vi "NIDCPower_channel_ganging - confgure triggers waveform mode.vi"(8 "error in (no error)":errorcluster, 11 "Ganged Session in":T1) -> (0 "error out":errorcluster, 3 "Ganged Session out":T1)   [LabVIEW 2021]
uses:
  ctl/NIDCPower_channel_ganging - ctl - channel mode.ctl
  <instrlib>/niDCPower/nidcpower.llb/niDCPower Configure Digital Edge Measure Trigger With Channels.vi
  <instrlib>/niDCPower/nidcpower.llb/niDCPower Configure Digital Edge Start Trigger With Channels.vi
  ctl/NIDCPower_channel_ganging - ctl - ganged config.ctl
  ctl/NIDCPower_channel_ganging - ctl - ganged session.ctl
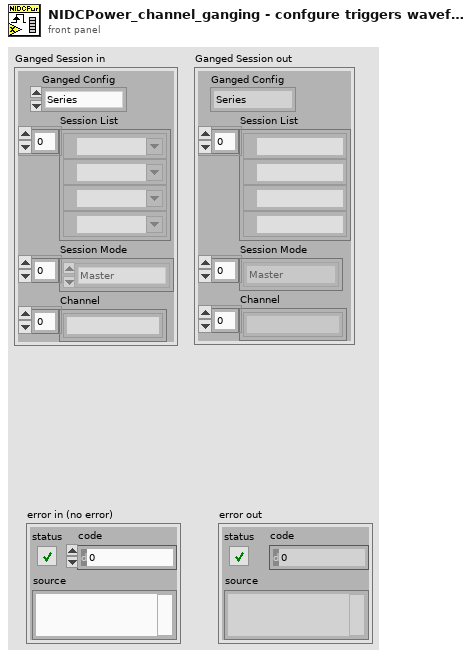
[diagram p1: front panel]
types:
  T1 = typedef "NIDCPower_channel_ganging - ctl - ganged session.ctl" = cluster{"Ganged Config":T2, "Session List":refnum<k15>[], "Session Mode":T3[], "Channel":string[]}
  T2 = typedef "NIDCPower_channel_ganging - ctl - ganged config.ctl" = enum16{"Series", "Parallel", "Manual"}
  T3 = typedef "NIDCPower_channel_ganging - ctl - channel mode.ctl" = enum16{"Master", "Slave", "Slave - Inverted"}
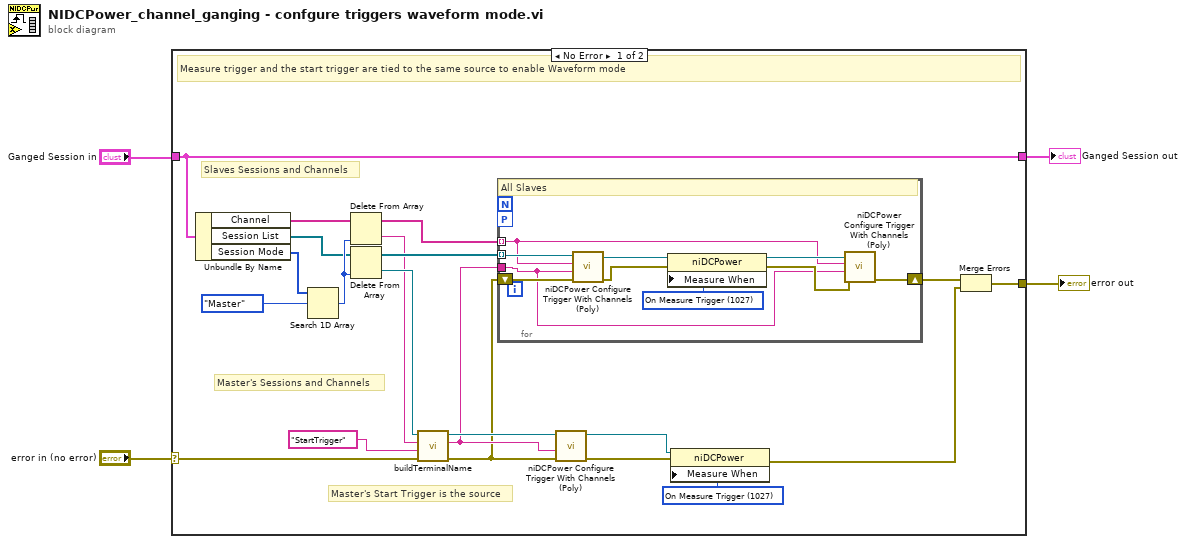
[diagram p0: block diagram]
diagram:
  n1 = case shown="No Error" "error in (no error)" {
    selector: "error in (no error)" -> [w23 w37]
    tunnel: [w9 w37] -> w4
    tunnel: "Ganged Session in" -> [w18 w36]
    tunnel: [w18 w36] -> w2
    frame No Error {
      w20 = 1027 items=["Automatically after Source Complete"=1025, "On Demand"=1026, "On Measure Trigger"=1027] ("Measurement:Advanced:Measure When")
      # "Master's Sessions and Channels"
      # "Slaves Sessions and Channels"
      # "Master's Start Trigger is the source"
      # "Measure trigger and the start trigger are tied to the same source to enable Waveform mode"
      n2 = Unbundle By Name(w18) -> ("Channel"=w14:string[], "Session List"=w13:refnum<k15>[], "Session Mode"=w6:T3[])
      n3 = Search 1D Array(1D array=w6, element=NIDCPower_channel_ganging_-_ctl_-_channel_mode."Master" ("Channel Mode")) -> (index of element=w16:i32)  [unwired: 1 in]
      n4 = Delete From Array(array=w14, index=w16) -> (deleted portion=w5:string, array with subset deleted=w15:string[])  [unwired: 1 in]
      n5 = Delete From Array(array=w13, index=w16) -> (deleted portion=w8:refnum<k15>, array with subset deleted=w17:refnum<k15>[])  [unwired: 1 in]
      n6 = call "buildTerminalName.vi"("error in (no error)"=w23, "Local Terminal Name"="StartTrigger" ("Trigger Type"), "Channel Name"=w5, "session handle"=w8) -> ("error out"=w7:errorcluster, "Fully Qualified Terminal Name"=w12:string, "session handle out"=w25:refnum<k15>)  [unwired: 5 in]
      n7 = for {
        tunnel: w15 -> [w27] mode=indexing
        tunnel: w17 -> [w28] mode=indexing
        shift-right: [w31] -> w11
        shift-left: w7 -> [w35]
        workers-P: _ -> [_]
        tunnel: w12 -> [w26]
        w32 = 1027 items=["Automatically after Source Complete"=1025, "On Demand"=1026, "On Measure Trigger"=1027] ("Measurement:Advanced:Measure When")
        # "All Slaves"
        n8 = call-poly <instrlib>:"niDCPower Configure Trigger With Channels (Poly).vi"("error in (no error)"=w35, "input terminal"=w26, "channel name"=w27, "instrument handle"=w28) -> ("error out"=w33:errorcluster, "instrument handle out"=w34:refnum<k15>)  [unwired: 6 in]
        n9 = property class="niDCPower"(reference=w34, error in=w33, "Measure When"=w32) -> (reference out=w30:refnum<k15>, error out=w29:errorcluster)
        n10 = call-poly <instrlib>:"niDCPower Configure Trigger With Channels (Poly).vi"("error in (no error)"=w29, "input terminal"=w26, "channel name"=w27, "instrument handle"=w30) -> ("error out"=w31:errorcluster)  [unwired: 6 in, 1 out]
      }
      n11 = call-poly <instrlib>:"niDCPower Configure Trigger With Channels (Poly).vi"("error in (no error)"=w7, "input terminal"=w12, "instrument handle"=w25) -> ("error out"=w22:errorcluster, "instrument handle out"=w21:refnum<k15>)  [unwired: 7 in]
      n12 = property class="niDCPower"(reference=w21, error in=w22, "Measure When"=w20) -> (error out=w10:errorcluster)  [unwired: 1 out]
      n13 = Merge Errors(w11, w10) -> (w9:errorcluster)
    }
    frame Error {
    }
  }
  "error out" <- w4
  "Ganged Session out" <- w2
